vi "Config IQ Adjustments.vi"(0 "VISA Resource Name":refnum<visa-resource-name>, 1 "I/Q Gain (0)":dbl format="%.2f", 2 "Quadrature Skew (0)":dbl format="%.2f", 5 "Status (T:ON)":bool=TRUE, 7 "I Offset (0)":dbl format="%.2f", 9 "Q Offset (0)":dbl format="%.2f", 11 "error in (no error)":errorcluster {"code" format="%.0x"}) -> (4 "VISA Resource Name Out":refnum<visa-resource-name>, 15 "error out":errorcluster {"code" format="%.0x"})   [LabVIEW 2014, in "Agilent ESG Series.lvlib"]
doc: "This VI is used to set the I/Q adjustments (I/Q Gain, I Offset ,Q Offset and Quadrature Skew).\n\nNotes:\n(1) This VI is for ESG-D and ESG-DP series only."
uses:
  Agilent ESG Series.lvlib
panel:
  # "ON"
  # "OFF"
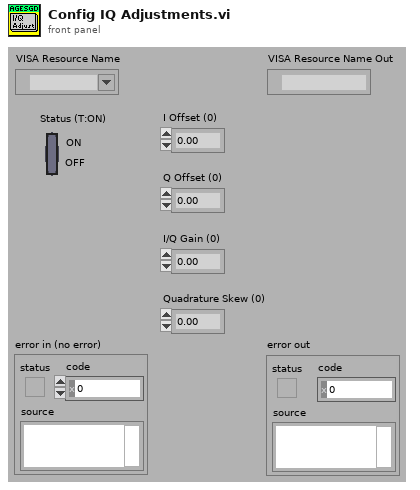
[diagram p1: front panel]
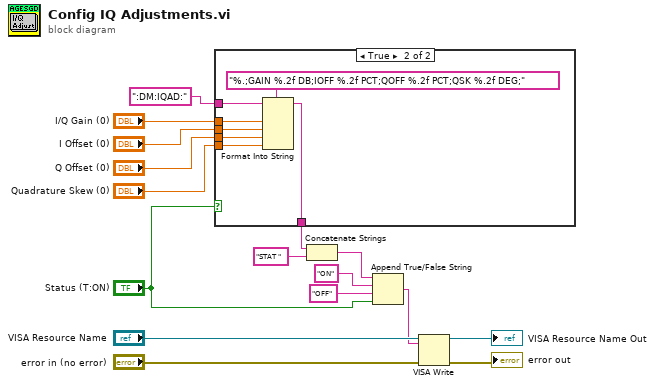
[diagram p0: block diagram]
diagram:
  n1 = case shown="True" "Status (T:ON)" {
    tunnel: "Quadrature Skew (0)" -> [_ w24]
    tunnel: "Q Offset (0)" -> [_ w23]
    tunnel: "I Offset (0)" -> [_ w22]
    tunnel: "I/Q Gain (0)" -> [_ w21]
    tunnel: [w17 w20] -> w7
    tunnel: ":DM:IQAD:" -> [w17 w18]
    frame False {
    }
    frame True {
      n2 = Format Into String(format string="%.;GAIN %.2f DB;IOFF %.2f PCT;QOFF %.2f PCT;QSK %.2f DEG;", initial string=w18, w21, w22, w23, w24) -> (resulting string=w20:string)  [unwired: 1 in, 1 out]
    }
  }
  n3 = Concatenate Strings(w7, "STAT ") -> (w11:string)
  n4 = Append True/False String(1:"Status (T:ON)", 2:"OFF" ("false string"), 3:"ON" ("true string"), 4:w11) -> (0:w1:string)
  n5 = VISA Write(VISA resource name="VISA Resource Name", write buffer=w1, error in (no error)="error in (no error)") -> (VISA resource name out=→"VISA Resource Name Out":refnum<visa-resource-name>, error out=→"error out":errorcluster)  [unwired: 1 out]
